vi "Set Moisture Level and Dither.vi"(11 "Error In":errorcluster) -> (15 "Error Out":errorcluster)   [LabVIEW 2016]
doc: "This VI gets or sets the GEA2 reference."
uses:
  <vilib>/DAQmx/write.llb/DAQmx Write (Analog DBL 1Chan 1Samp).vi
  <vilib>/DAQmx/create/channels.llb/DAQmx Create Channel (AO-Voltage-Basic).vi
  <vilib>/DAQmx/miscellaneous.llb/DAQmx Fill In Error Info.vi
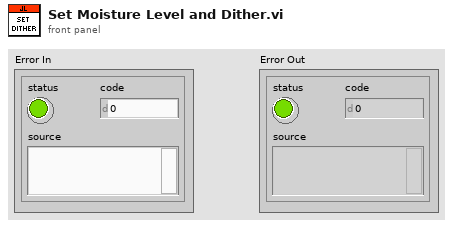
[diagram p1: front panel]
types:
  T1 = typedef "Moisture Data.ctl" = cluster{"Moisture (V)":dbl, "Dither":dbl, "Stop":bool}
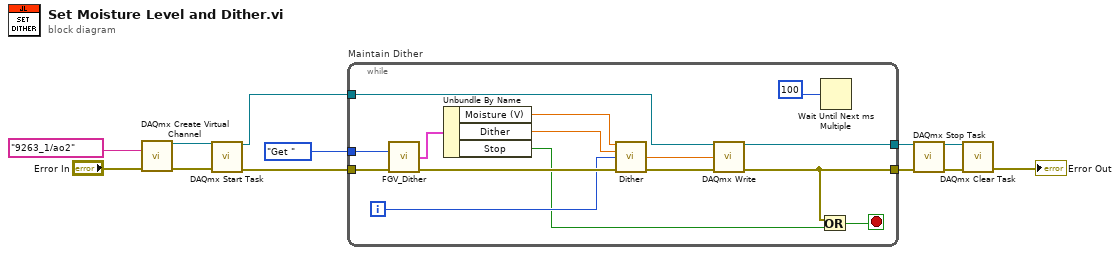
[diagram p0: block diagram]
diagram:
  n1 = call-poly <vilib>:"DAQmx Create Virtual Channel.vi"("physical channels"=tag "9263_1/ao2", "error in"="Error In") -> ("task out"=w8:refnum<k21>, "error out"=w7:errorcluster)  [unwired: 12 in]
  n2 = call <vilib>:"DAQmx Start Task.vi"("task/channels in"=w8, "error in"=w7) -> ("task out"=w3:refnum<k21>, "error out"=w5:errorcluster)  [unwired: 12 in]
  n3 = while "Maintain Dither" {
    tunnel: [w15] -> w9
    tunnel: w5 -> [w26]
    tunnel: enum16{"Set", "Get "}."Get " ("Action") -> [w16]
    tunnel: [w18] -> w4
    tunnel: w3 -> [w17]
    i -> [w23]
    stop <- w14 stop-if-true
    n4 = call "FGV_Dither.vi"("Action"=w16, "Error In"=w26) -> ("Moisture Data Out"=w24:T1, "Error Out"=w25:errorcluster)  [unwired: 12 in]
    n5 = Unbundle By Name(w24) -> ("Moisture (V)"=w19:dbl, "Dither"=w20:dbl, "Stop"=w13:bool)
    n6 = call "Dither.vi"("Moisture (V) in"=w19, "Dither"=w20, "Iteration Terminal"=w23, "Error In"=w25) -> ("Moisture (V)"=w27:dbl, "Error Out"=w22:errorcluster)  [unwired: 10 in]
    n7 = call-poly <vilib>:"DAQmx Write.vi"("task/channels in"=w17, "data"=w27, "error in"=w22) -> ("task out"=w18:refnum<k21>, "error out"=w15:errorcluster)  [unwired: 10 in, 1 out]
    n8 = Or(x=w15, y=w13) -> (x .or. y?=w14:bool)
    n9 = Wait Until Next ms Multiple(millisecond multiple=u32 100) -> ()  [unwired: 1 out]
  }
  n10 = call <vilib>:"DAQmx Stop Task.vi"("task/channels in"=w4, "error in"=w9) -> ("task out"=w11:refnum<k21>, "error out"=w12:errorcluster)  [unwired: 12 in]
  n11 = call <vilib>:"DAQmx Clear Task.vi"("task in"=w11, "error in"=w12) -> ("error out"=→"Error Out":errorcluster)  [unwired: 13 in]
